vi "Befehl senden Amium.vi"(11 "connection ID":refnum<k5>) -> (0 "error out":errorcluster, 2 "Verknüpfter String":string, 3 "connection ID":refnum<k5>)   [LabVIEW 2020, in "Amium PNS.lvlib" / "AK Kommunikation.lvlib"]
uses:
  AK Kommunikation.lvlib
  Amium Kommandos verwalten Aktionen.ctl
  TCP Timeout Aktionen - Amium.ctl
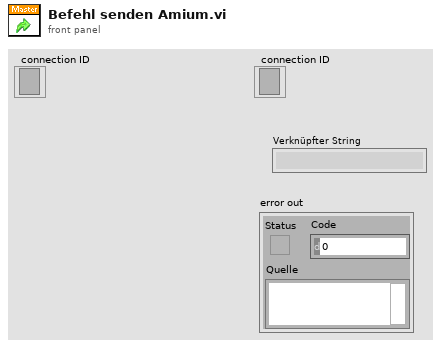
[diagram p1: front panel]
types:
  T1 = typedef "Amium PNS.lvlib/AK Kommunikation.lvlib/TCP Timeout Aktionen - Amium.ctl" = enum16{"lesen", "setzen"}
  T2 = typedef "Amium PNS.lvlib/AK Kommunikation.lvlib/Amium Kommandos verwalten Aktionen.ctl" = enum16{"lesen", "setzen Ende", "setzen Pos1", "senden", "initalisieren", "prüfen", "Kommandos"}
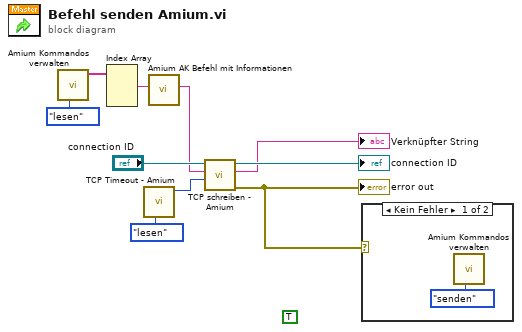
[diagram p0: block diagram]
diagram:
  (unwired) TRUE
  n1 = call "Amium Kommandos verwalten.vi"("Aktionen"=Amium_Kommandos_verwalten_Aktionen."lesen") -> ("Kommandos"=w4:string[])  [unwired: 8 in, 2 out]
  n2 = Index Array(array=w4) -> (element #1=w6:string)  [unwired: 3 in, 2 out]
  n3 = call "TCP Timeout - Amium.vi"("Aktionen Timeout"=TCP_Timeout_Aktionen_-_Amium."lesen") -> ("Timeout schreiben"=w3:i32)  [unwired: 9 in, 1 out]
  n4 = call "Amium AK Befehl mit Informationen.vi"("AK Befehl"=w6) -> ("String für schreiben"=w5:string)  [unwired: 10 in]
  n5 = call "TCP schreiben - Amium.vi"("Timeout schreiben"=w3, "String"=w5, "connection ID"="connection ID") -> ("error out"=w9:errorcluster, "Verknüpfter String"=→"Verknüpfter String":string, "connection ID"=→"connection ID":refnum<k5>)  [unwired: 6 in]
  "error out" <- w9
  n6 = case shown="Kein Fehler" w9 {
    frame No Error {
      n7 = call "Amium Kommandos verwalten.vi"("Aktionen"=Amium_Kommandos_verwalten_Aktionen."senden") -> ()  [unwired: 8 in, 3 out]
    }
    frame Error {
    }
  }
